vi "setWavelength.vi"(8 "error in (no error)":errorcluster, 9 "Monochromator in":refnum<class "Monochromator.lvclass">, 10 "wavelength":T1, 11 "ReadySate in":refnum<class "ReadySate.lvclass">) -> (0 "error out":errorcluster, 1 "Monochromator out":refnum<class "Monochromator.lvclass">, 3 "ReadySate out":refnum<class "ReadySate.lvclass">)   [LabVIEW 2016, in "ReadySate.lvclass"]
uses:
  ReadySate.lvclass
  Typedefs/wavelength.ctl
  Monochromator/Monochromator.lvclass
  Typedefs/SWStatus.ctl
  Typedefs/AckType.ctl
  Monochromator/Monochromator.lvclass/Monochromator.ctl
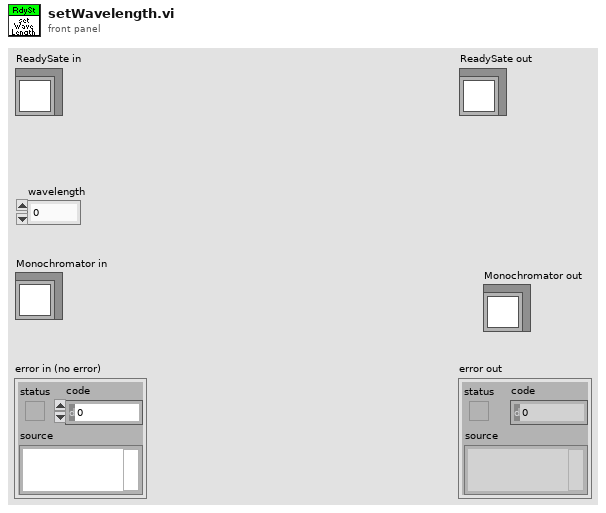
[diagram p1: front panel]
types:
  T1 = typedef "wavelength.ctl" = dbl
  T2 = typedef "AckType.ctl" = enum16{"OK", "OutOfRange", "Unknown", "Busy", "Rejected"}
  T3 = typedef "SWStatus.ctl" = enum16{"OfflineState", "ReadyState", "SettingUpState", "FaultState"}
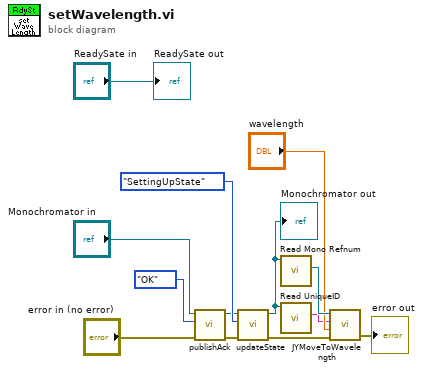
[diagram p0: block diagram]
diagram:
  n1 = call "publishAck.vi"("error in (no error)"="error in (no error)", "Ack"=AckType."OK" ("AckType"), "Monochromator in"="Monochromator in") -> ("error out"=w5:errorcluster, "Monochromator out"=w4:refnum<class "Monochromator.lvclass">)  [unwired: 7 in]
  n2 = call "updateState.vi"("error in (no error)"=w5, "SWStatus"=SWStatus."SettingUpState", "Monochromator in"=w4) -> ("error out"=w7:errorcluster, "Monochromator out"=w6:refnum<class "Monochromator.lvclass">)  [unwired: 7 in]
  "Monochromator out" <- w6
  n3 = call "Read Mono Refnum.vi"("Monochromator in"=w6) -> ("Mono Refnum"=w13:refnum<k7>)  [unwired: 8 in, 2 out]
  n4 = call "Read UniqueID.vi"("Monochromator in"=w6) -> ("UniqueID"=w10:string)  [unwired: 8 in, 2 out]
  n5 = call "JYMoveToWavelength.vi"("error in (no error)"=w7, "Target WL"="wavelength", "UniqueID"=w10, "RefNum In"=w13) -> ("error out"=→"error out":errorcluster)  [unwired: 2 out]
  "ReadySate out" <- "ReadySate in"
